vi "Work Sheet Referrence.vi"(8 "error in":errorcluster, 10 "Sheet Name":string, 11 "Worksheets 2":refnum<k7>) -> (0 "error out":errorcluster, 1 "Work Sheet":refnum<k7>, 2 "Worksheets":refnum<k7>)   [LabVIEW 2017]
panel:
  out "Name":string
  in  "Excel._Worksheet":refnum<k7>
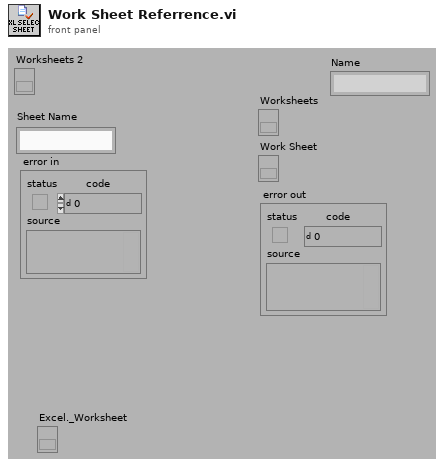
[diagram p1: front panel]
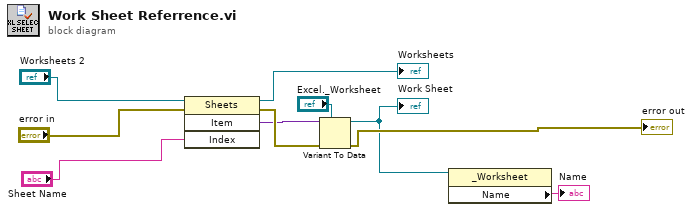
[diagram p0: block diagram]
diagram:
  n1 = invoke class="Sheets" method="Item"(reference="Worksheets 2", error in="error in", "Index"="Sheet Name") -> (reference out=→"Worksheets":refnum<k7>, error out=w10:errorcluster, "Item"=w6:variant)  [unwired: 1 in, 1 out]
  n2 = Variant To Data(error in=w10, type="Excel._Worksheet", Variant=w6) -> (data=w2:refnum<k7>, error out=→"error out":errorcluster)
  "Work Sheet" <- w2
  n3 = property class="_Worksheet"(reference=w2) -> ("Name"=→"Name":string)  [unwired: 1 in, 2 out]
